vi "GV Nmax pixel clock.vi"() -> ()   [LabVIEW 2017]
panel:
  out "Nmax pixel clock":u16
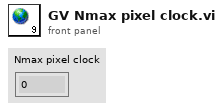
[diagram p1: front panel]
diagram:
